vi "test30-MappingRelationshipByLocalRegistration_WIthSubscriberName_State.vi"(8 "error in (no error)":errorcluster, 11 "TestCase in":refnum<class "testcase-CSMBroadcast.lvclass">) -> (0 "error out":errorcluster, 3 "TestCase out":refnum<class "testcase-CSMBroadcast.lvclass">)   [LabVIEW 2017, in "testcase-CSMBroadcast.lvclass"]
uses:
  testcase-CSMBroadcast.lvclass
  caa41fc0-4920-4570-a7eb-0567c3b7bd6c.vi
  <vilib>/addons/_JKI Toolkits/VI Tester/TestCase.llb/TestCase.lvclass
  src/user.lib/_NEVSTOP/Communicable State Machine(CSM)/Communicable State Machine.lvlib
  CSM/CSM-Testcase.lvlib
  C:/Program Files (x86)/National Instruments/LabVIEW 2017/vi.lib/addons/_JKI Toolkits/VI Tester/TestCase.llb/TestCase.lvclass
panel:
  out "Loop Count":i32
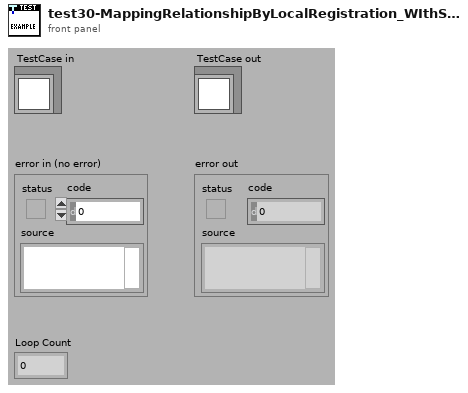
[diagram p1: front panel]
types:
  T1 = cluster{"Status":string, "Source CSM":string, "Target CSM":string, "Target API":string}[]
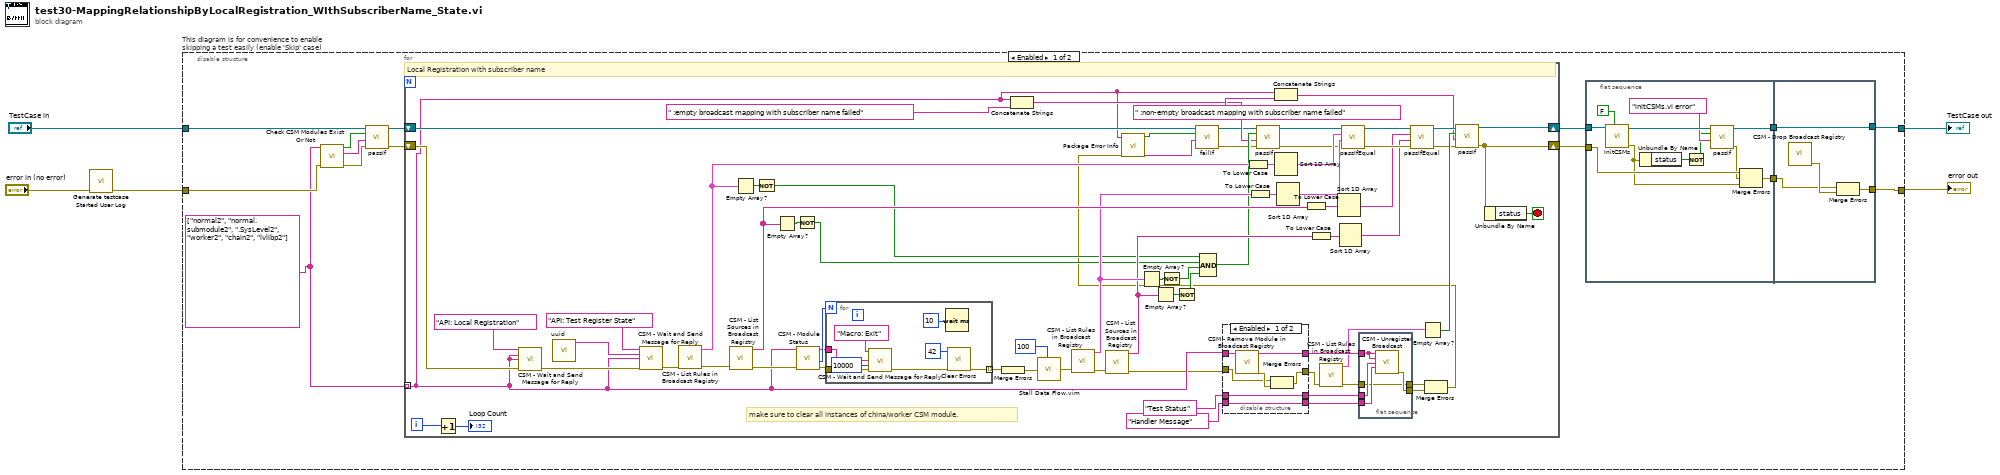
[diagram p0: block diagram]
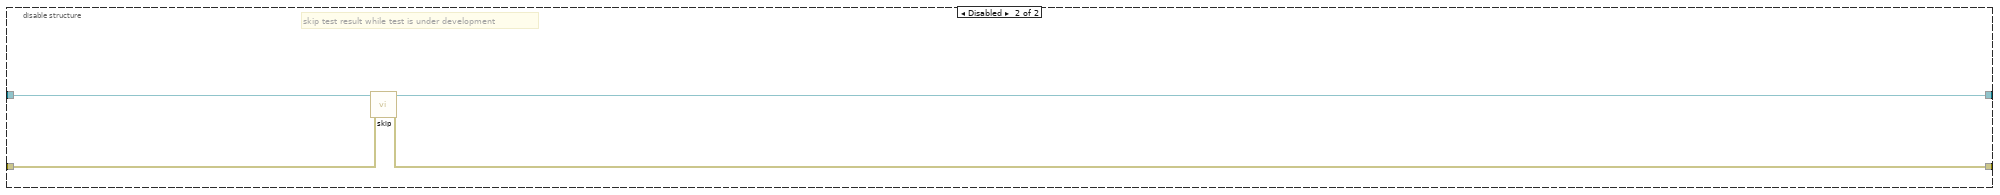
[diagram p3: hidden frame]
diagram:
  n1 = call "Generate testcase Started User Log.vi"("Error In"="error in (no error)") -> ("error out"=w1:errorcluster)  [unwired: 10 in]
  n2 = disable-structure "This diagram is for convenience to enable skipping a test easily (enable 'Skip' case)" shown="Enabled" {
    disable-tunnel: "TestCase in" -> [w16 w133]
    disable-tunnel: [w8 w131] -> w2
    disable-tunnel: [w7 w132] -> w4
    disable-tunnel: w1 -> [w14 w130]
    frame Enabled {
      w6 = string[] ["normal2", "normal.submodule2", ".SysLevel2", "worker2", "chain2", "lvlibp2"]
      n3 = call "Check CSM Modules Exist Or Not.vi"("error in"=w14, "CSM names in"=w6) -> ("error out"=w17:errorcluster, "Debug string"=w18:string, "All Modules Exist?"=w19:bool)  [unwired: 7 in]
      n4 = call-dynamic "passIf.vi"("error in (no error)"=w17, "message (\"\")"=w18, "pass"=w19, "TestCase in"=w16) -> ("error out"=w13:errorcluster, "TestCase out"=w15:refnum<class "testcase-CSMBroadcast.lvclass">)  [unwired: 6 in]
      n5 = for {
        tunnel: w6 -> [w40] mode=indexing
        shift-right: [w70] -> w10
        shift-left: w15 -> [w51]
        shift-right: [w71] -> w9
        shift-left: w13 -> [w61]
        i -> [w86]
        stop <- w99 stop-if-true
        # "make sure to clear all instances of china/worker CSM module."
        # "Local Registration with subscriber name"
        n6 = Increment(x=w86) -> (x+1=→"Loop Count":i32)
        n7 = call "CSM - Wait and Send Message for Reply.vi"("State"="API: Local Registration", "Arguments (\"\")"=w40, "Target Module"=w40, "Error In (No Error)"=w61) -> ("error out"=w104:errorcluster)  [unwired: 8 in, 3 out]
        n8 = call "uuid.vi"() -> ("UUID"=w102:string)  [unwired: 11 in]
        n9 = call "CSM - Wait and Send Message for Reply.vi"("State"="API: Test Register State", "Arguments (\"\")"=w102, "Target Module"=w40, "Error In (No Error)"=w104) -> ("error out"=w101:errorcluster)  [unwired: 8 in, 3 out]
        n10 = call "CSM - List Rules in Broadcast Registry.vi"("error in (no error)"=w101) -> ("error out"=w98:errorcluster, "Rule Entries"=w84:T1)  [unwired: 8 in, 1 out]
        n11 = call "CSM - List Sources in Broadcast Registry.vi"("error in (no error)"=w98) -> ("error out"=w66:errorcluster, "Broadcast Names"=w81:string[])  [unwired: 9 in]
        n12 = Empty Array?(array=w84) -> (empty?=w83:bool)
        n13 = Not(x=w83) -> (.not. x?=w76:bool)
        n14 = Empty Array?(array=w81) -> (empty?=w82:bool)
        n15 = Not(x=w82) -> (.not. x?=w75:bool)
        n16 = call "CSM - Module Status.vi"("Error In"=w66, "CSM Name"=w40) -> ("error out"=w67:errorcluster, "#Nodes"=w69:i32, "CSM Name (Dup)"=w68:string)  [unwired: 5 in, 2 out]
        n17 = for {
          N: w69 -> [_]
          tunnel: w68 -> [w128]
          tunnel: w67 -> [w127]
          tunnel: [w124] -> w100 mode=indexing
          n18 = call "CSM - Wait and Send Message for Reply.vi"("State"="Macro: Exit", "Target Module"=w128, "Wait (5000ms)"=10000, "Error In (No Error)"=w127) -> ("error out"=w125:errorcluster)  [unwired: 8 in, 3 out]
          n19 = Wait (ms)(milliseconds to wait=u32 10) -> ()  [unwired: 1 out]
          n20 = call <vilib>:"Clear Errors.vi"("error in (no error)"=w125, "specific error code to clear (0: all)"=42) -> ("error out"=w124:errorcluster)  [unwired: 4 in, 1 out]
        }
        n21 = Merge Errors(w100) -> (w55:errorcluster)
        n22 = Concatenate Strings(w40, " :empty broadcast mapping with subscriber name failed" ("string")) -> (w57:string)
        n23 = call "Stall Data Flow.vim"("value in"=w55, "milliseconds to wait"=u32 100) -> ("value out"=w54:errorcluster)  [unwired: 1 out]
        n24 = call "CSM - List Rules in Broadcast Registry.vi"("error in (no error)"=w54) -> ("error out"=w97:errorcluster, "Rule Entries"=w79:T1)  [unwired: 8 in, 1 out]
        n25 = call "CSM - List Sources in Broadcast Registry.vi"("error in (no error)"=w97) -> ("error out"=w37:errorcluster, "Broadcast Names"=w77:string[])  [unwired: 9 in]
        n26 = Empty Array?(array=w79) -> (empty?=w80:bool)
        n27 = Empty Array?(array=w77) -> (empty?=w78:bool)
        n28 = Not(x=w80) -> (.not. x?=w74:bool)
        n29 = Not(x=w78) -> (.not. x?=w73:bool)
        n30 = Compound Arithmetic op=AND(w76, w75, w74, w73) -> (w60:bool)
        n31 = disable-structure shown="Enabled" {
          disable-tunnel: w37 -> [w111 w120]
          disable-tunnel: [w115 w120] -> w46
          disable-tunnel: w40 -> [w116 w121]
          disable-tunnel: "Test Status" ("Status") -> [w113 w119]
          disable-tunnel: "Handler Message" ("Response Message (If \"\", Same as Source Message)") -> [w112 w118]
          disable-tunnel: [w114 w121] -> w47
          disable-tunnel: [w113 w119] -> w45
          disable-tunnel: [w112 w118] -> w44
          frame Enabled {
            n32 = call "CSM - Remove Module in Broadcast Registry.vi"("CSM Name"=w116) -> ("CSM Name (Dup)"=w114:string, "error out"=w117:errorcluster)  [unwired: 13 in]
            n33 = Merge Errors(w111, w117) -> (w115:errorcluster)
          }
          frame Disabled {
          }
        }
        n34 = To Lower Case(string=w84) -> (all lower case string=w96:T1)
        n35 = To Lower Case(string=w79) -> (all lower case string=w95:T1)
        n36 = Concatenate Strings(w40, " :non-empty broadcast mapping with subscriber name failed" ("string")) -> (w56:string)
        n37 = Sort 1D Array(array=w96) -> (sorted array=w94:T1)
        n38 = Sort 1D Array(array=w95) -> (sorted array=w93:T1)
        n39 = To Lower Case(string=w81) -> (all lower case string=w90:string[])
        n40 = To Lower Case(string=w77) -> (all lower case string=w89:string[])
        n41 = call "CSM - List Rules in Broadcast Registry.vi"("error in (no error)"=w46) -> ("error out"=w42:errorcluster, "Rule Entries"=w39:T1)  [unwired: 8 in, 1 out]
        n42 = Sort 1D Array(array=w90) -> (sorted array=w88:string[])
        n43 = Sort 1D Array(array=w89) -> (sorted array=w87:string[])
        n44 = flat-sequence {
          tunnel: w47 -> [w110]
          tunnel: w45 -> [w109]
          tunnel: w44 -> [w108]
          tunnel: [w107] -> w43
          tunnel: w42 -> [w106]
          tunnel: [w106] -> w41
          frame #0 {
            n45 = call "CSM - Unregister Broadcast.vi"("CSM Name(Empty for Broadcast Event)"=w110, "Source CSM Name (* as Default)"=w110, "Trigger"=w109, "API (\"*\" as Default)"=w108) -> ("error out"=w107:errorcluster)  [unwired: 10 in, 1 out]
          }
        }
        n46 = Empty Array?(array=w39) -> (empty?=w72:bool)
        n47 = Merge Errors(w41, w43) -> (w38:errorcluster)
        n48 = call "Package Error Info.vi"("error in"=w38, "String in"=w40) -> ("packed error info out"=w48:string, "error status"=w49:bool)  [unwired: 8 in]
        n49 = call-dynamic "failIf.vi"("message (\"\")"=w48, "fail"=w49, "TestCase in"=w51) -> ("error out"=w50:errorcluster, "TestCase out"=w52:refnum<class "testcase-CSMBroadcast.lvclass">)  [unwired: 7 in]
        n50 = call-dynamic "passIf.vi"("error in (no error)"=w50, "message (\"\")"=w57, "pass"=w60, "TestCase in"=w52) -> ("error out"=w62:errorcluster, "TestCase out"=w63:refnum<class "testcase-CSMBroadcast.lvclass">)  [unwired: 6 in]
        n51 = call-dynamic "passIfEqual.vi"("error in (no error)"=w62, "y"=w93, "x"=w94, "TestCase in"=w63) -> ("error out"=w91:errorcluster, "TestCase out"=w92:refnum<class "testcase-CSMBroadcast.lvclass">)  [unwired: 6 in]
        n52 = call-dynamic "passIfEqual.vi"("error in (no error)"=w91, "y"=w87, "x"=w88, "TestCase in"=w92) -> ("error out"=w64:errorcluster, "TestCase out"=w65:refnum<class "testcase-CSMBroadcast.lvclass">)  [unwired: 6 in]
        n53 = call-dynamic "passIf.vi"("error in (no error)"=w64, "message (\"\")"=w56, "pass"=w72, "TestCase in"=w65) -> ("error out"=w71:errorcluster, "TestCase out"=w70:refnum<class "testcase-CSMBroadcast.lvclass">)  [unwired: 6 in]
        n54 = Unbundle By Name(w71) -> ("status"=w99:bool)
      }
      n55 = flat-sequence {
        tunnel: w10 -> [w30]
        tunnel: [w27] -> w12
        tunnel: w9 -> [w24]
        tunnel: [w21] -> w11
        tunnel: w12 -> [w33]
        tunnel: [w33] -> w8
        tunnel: [w32] -> w7
        tunnel: w11 -> [w31]
        frame #0 {
          n56 = call "InitCSMs.vi"("Enable building lvlibp?"=FALSE, "testcase-CSMStatus in"=w30) -> ("error out"=w22:errorcluster, "testcase-CSMStatus out"=w28:refnum<class "testcase-CSMBroadcast.lvclass">)  [unwired: 8 in]
          n57 = Unbundle By Name(w22) -> ("status"=w26:bool)
          n58 = Not(x=w26) -> (.not. x?=w20:bool)
          n59 = call-dynamic "passIf.vi"("message (\"\")"="initCSMs.vi error" ("message (\"\")"), "pass"=w20, "TestCase in"=w28) -> ("error out"=w23:errorcluster, "TestCase out"=w27:refnum<class "testcase-CSMBroadcast.lvclass">)  [unwired: 7 in]
          n60 = Merge Errors(w24, w23, w22) -> (w21:errorcluster)
        }
        frame #1 {
          n61 = call "CSM - Drop Broadcast Registry.vi"() -> ("error out"=w34:errorcluster)  [unwired: 15 in]
          n62 = Merge Errors(w31, w34) -> (w32:errorcluster)
        }
      }
    }
    frame Disabled {
      # "skip test result while test is under development"
      n63 = call <vilib>:"skip.vi"("error in (no error)"=w130, "TestCase in"=w133) -> ("error out"=w132:errorcluster, "TestCase out"=w131:refnum<class "testcase-CSMBroadcast.lvclass">)  [unwired: 8 in]
    }
  }
  "error out" <- w4
  "TestCase out" <- w2
